vi "removeDPScript.vi"(8 "error in (no error)":errorcluster, 11 "ExperimentRunner in":refnum<class "ExperimentRunner.lvclass">) -> (0 "error out":errorcluster, 3 "ExperimentRunner out":refnum<class "ExperimentRunner.lvclass">)   [LabVIEW 2009, in "Views.lvlib" / "ExperimentControl.lvlib" / "ExperimentRunner.lvclass"]
doc: "Removes a script path from the path array"
uses:
  ExperimentRunner.lvclass
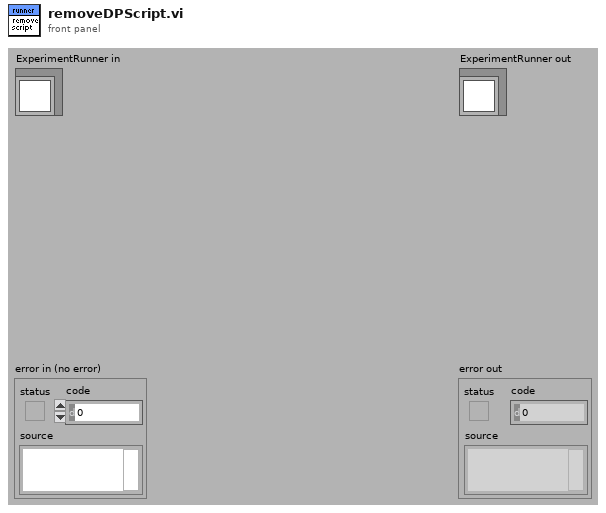
[diagram p1: front panel]
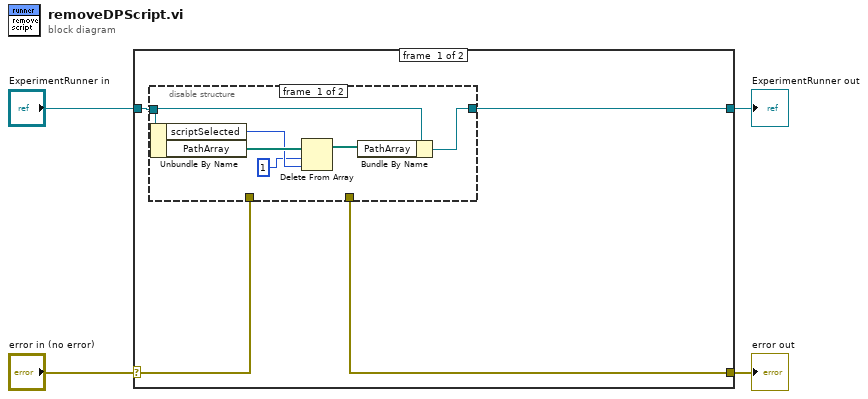
[diagram p0: block diagram]
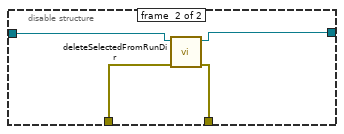
[diagram p2: hidden frame]
diagram:
  n1 = case shown="No Error" "error in (no error)" {
    selector: "error in (no error)" -> [w6 w20]
    tunnel: [w5 w20] -> w3
    tunnel: [w7 w19] -> w1
    tunnel: "ExperimentRunner in" -> [w8 w19]
    frame #0 {
      n2 = disable-structure shown="Enabled" {
        disable-tunnel: w8 -> [w11 w18]
        disable-tunnel: [w10 w17] -> w7
        disable-tunnel: w6 -> [_ w16]
        disable-tunnel: [_ w15] -> w5
        frame #0 {
          n3 = Unbundle By Name(w11) -> ("scriptSelected"=w13:i32, "PathArray"=w14:path[])
          n4 = Delete From Array(array=w14, length=1, index=w13) -> (array with subset deleted=w9:path[])  [unwired: 1 out]
          n5 = Bundle By Name(cluster=w11, "PathArray"=w9) -> (w10:refnum<class "ExperimentRunner.lvclass">)
        }
        frame #1 {
          n6 = call "deleteSelectedFromRunDir.vi"("error in (no error)"=w16, "ExperimentRunner in"=w18) -> ("error out"=w15:errorcluster, "ExperimentRunner out"=w17:refnum<class "ExperimentRunner.lvclass">)  [unwired: 8 in]
        }
      }
    }
    frame #1 {
    }
  }
  "error out" <- w3
  "ExperimentRunner out" <- w1
